vi "FdxCmdBoardControlCvi.vi"(8 "error in":errorcluster, 9 "BoardControlIn (read)":T4 {"Expert4Mode" items=["FDX_EXPERT_MODE", "FDX_DISA_GHOST"]; "Expert3Mode" items=["FDX_EXPERT_MODE", "FDX_DISA_GHOST"]; "Expert2Mode" items=["FDX_EXPERT_MODE", "FDX_DISA_GHOST"]; "Expert1Mode" items=["FDX_EXPERT_MODE", "FDX_DISA_GHOST"]; "Port4SpeedIn" items=["FDX_100MBIT", "FDX_10MBIT", "FDX_AUTO_100MBIT", "FDX_AUTO_10MBIT"]; "Port3SpeedIn" items=["FDX_100MBIT", "FDX_10MBIT", "FDX_AUTO_100MBIT", "FDX_AUTO_10MBIT"]; "Port2SpeedIn" items=["FDX_100MBIT", "FDX_10MBIT", "FDX_AUTO_100MBIT", "FDX_AUTO_10MBIT"]; "Port1SpeedIn" items=["FDX_100MBIT", "FDX_10MBIT", "FDX_AUTO_100MBIT", "FDX_AUTO_10MBIT"]; "Port4ConfigIn" items=["FDX_SINGLE", "FDX_REDUNDANT"]; "Port3ConfigIn" items=["FDX_SINGLE", "FDX_REDUNDANT"]; "Port2ConfigIn" items=["FDX_SINGLE", "FDX_REDUNDANT"]; "Port1ConfigIn" items=["FDX_SINGLE", "FDX_REDUNDANT"]; "Control" items=["FDX_READ", "FDX_WRITE"]}, 11 "InstrumentHandle_board in":u32) -> (0 "error out":errorcluster, 1 "Board Control Out":T6 {"SharedMemFree" format="%x"; "GlobalMemFree" format="%x"; "ExpertMode" items=["FDX_EXPERT_MODE", "FDX_DISA_GHOST"]; "PortGoodLink" items=["FDX_NO_LINK", "FDX_GOOD_LINK"]; "PortSpeed" items=["FDX_100MBIT", "FDX_10MBIT", "FDX_AUTO_100MBIT", "FDX_AUTO_10MBIT"]; "PortConfig" items=["FDX_SINGLE", "FDX_REDUNDANT"]}, 3 "InstrumentHandle_board out":u32)   [LabVIEW 2020, in "AIM664LV.lvlib"]
doc: "This function is used to control the global settings of the board. For the AIM-FDX board this means the organization of the physical ports to logical single or redundant ports."
uses:
  AIM664LV.lvlib
  _controls/port_configuration.ctl
  _controls/port_speed.ctl
  _controls/port_condition.ctl
  _controls/expert_mode.ctl
  AFDX_LibraryAdmin/FdxGlobalDllPath.vi
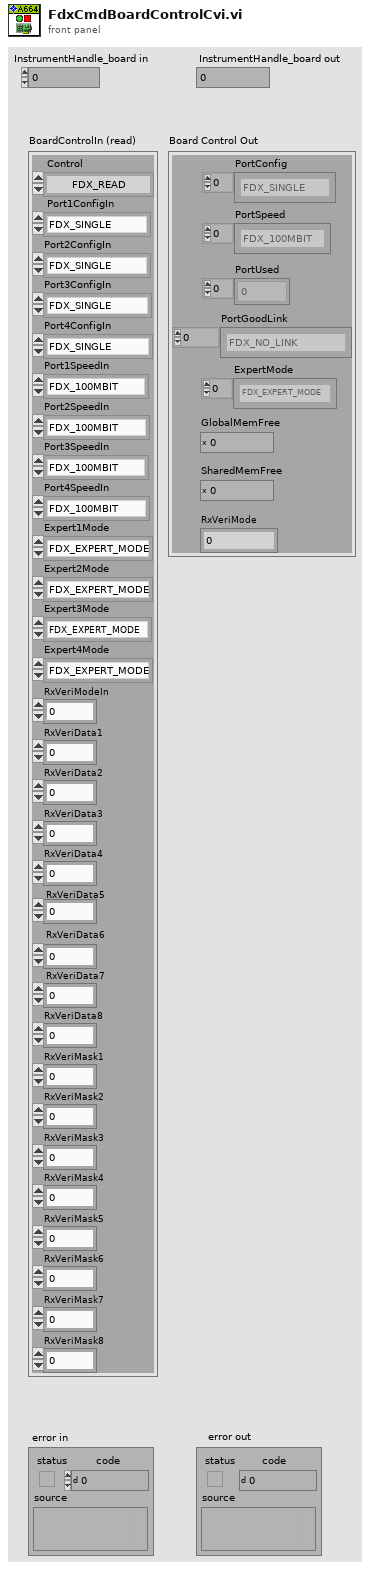
[diagram p1: front panel]
types:
  T1 = typedef "AIM664LV.lvlib/port_configuration.ctl" = u32
  T2 = typedef "AIM664LV.lvlib/port_speed.ctl" = u32
  T3 = typedef "AIM664LV.lvlib/expert_mode.ctl" = u32
  T4 = cluster{"Control":u32, "Port1ConfigIn":T1, "Port2ConfigIn":T1, "Port3ConfigIn":T1, "Port4ConfigIn":T1, "Port1SpeedIn":T2, "Port2SpeedIn":T2, "Port3SpeedIn":T2, "Port4SpeedIn":T2, "Expert1Mode":T3, "Expert2Mode":T3, "Expert3Mode":T3, "Expert4Mode":T3, "RxVeriModeIn":u32, "RxVeriData1":u32, "RxVeriData2":u32, "RxVeriData3":u32, "RxVeriData4":u32, "RxVeriData5":u32, "RxVeriData6":u32, "RxVeriData7":u32, "RxVeriData8":u32, "RxVeriMask1":u32, "RxVeriMask2":u32, "RxVeriMask3":u32, "RxVeriMask4":u32, "RxVeriMask5":u32, "RxVeriMask6":u32, "RxVeriMask7":u32, "RxVeriMask8":u32}
  T5 = typedef "AIM664LV.lvlib/port_condition.ctl" = u32
  T6 = cluster{"PortConfig":T1[], "PortSpeed":T2[], "PortUsed":u32[], "PortGoodLink":T5[], "ExpertMode":T3[], "GlobalMemFree":u32, "SharedMemFree":u32, "RxVeriMode":u32}
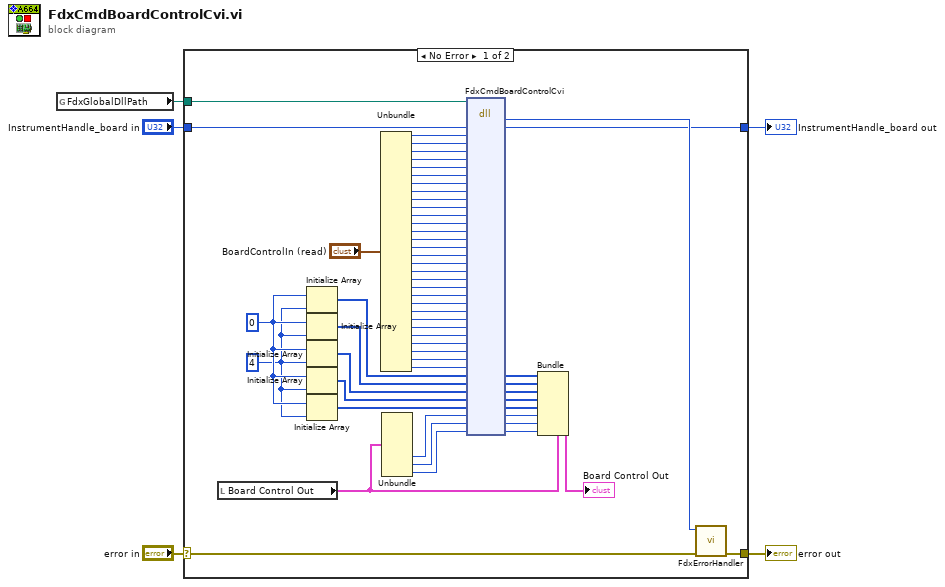
[diagram p0: block diagram]
diagram:
  n1 = global read "FdxGlobalDllPath.vi" "FdxGlobalDllPath"() -> (w3:path)
  n2 = case shown="No Error" "error in" {
    selector: "error in" -> [w62 w64]
    tunnel: [w61 w64] -> w5
    tunnel: w3 -> [w8 _]
    tunnel: "InstrumentHandle_board in" -> [w7 w63]
    tunnel: [w6 w63] -> w1
    frame No Error {
      w49 = 4
      w50 = u32 0
      n3 = local read "Board Control Out"() -> (w9:T6)
      n4 = Initialize Array(w50, w49) -> (w40:u32[])
      n5 = Initialize Array(w50, w49) -> (w39:u32[])
      n6 = Initialize Array(w50, w49) -> (w38:u32[])
      n7 = Initialize Array(w50, w49) -> (w37:u32[])
      n8 = Initialize Array(w50, w49) -> (w36:u32[])
      n9 = Unbundle("BoardControlIn (read)") -> ("Control"=w59:u32, "Port1ConfigIn"=w58:T1, "Port2ConfigIn"=w57:T1, "Port3ConfigIn"=w56:T1, "Port4ConfigIn"=w55:T1, "Port1SpeedIn"=w54:T2, "Port2SpeedIn"=w53:T2, "Port3SpeedIn"=w52:T2, "Port4SpeedIn"=w51:T2, "Expert1Mode"=w48:T3, "Expert2Mode"=w47:T3, "Expert3Mode"=w46:T3, "Expert4Mode"=w41:T3, "RxVeriModeIn"=w44:u32, "RxVeriData1"=w43:u32, "RxVeriData2"=w42:u32, "RxVeriData3"=w29:u32, "RxVeriData4"=w28:u32, "RxVeriData5"=w27:u32, "RxVeriData6"=w26:u32, "RxVeriData7"=w25:u32, "RxVeriData8"=w24:u32, "RxVeriMask1"=w23:u32, "RxVeriMask2"=w22:u32, "RxVeriMask3"=w21:u32, "RxVeriMask4"=w20:u32, "RxVeriMask5"=w19:u32, "RxVeriMask6"=w18:u32, "RxVeriMask7"=w17:u32, "RxVeriMask8"=w16:u32)
      n10 = Unbundle(w9) -> ("GlobalMemFree"=w15:u32, "SharedMemFree"=w14:u32, "RxVeriMode"=w13:u32)  [unwired: 5 out]
      n11 = dll-call lib="aim_fdx.19.dll" fn="FdxCmdBoardControlCvi"(path in=w8, "InstrumentHandle"=w7, "Control"=w59, "Port1ConfigIn"=w58, "Port2ConfigIn"=w57, "Port3ConfigIn"=w56, "Port4ConfigIn"=w55, "Port1SpeedIn"=w54, "Port2SpeedIn"=w53, "Port3SpeedIn"=w52, "Port4SpeedIn"=w51, "Expert1Mode"=w48, "Expert2Mode"=w47, "Expert3Mode"=w46, "Expert4Mode"=w41, "RxVeriModeIn"=w44, "RxVeriData1"=w43, "RxVeriData2"=w42, "RxVeriData3"=w29, "RxVeriData4"=w28, "RxVeriData5"=w27, "RxVeriData6"=w26, "RxVeriData7"=w25, "RxVeriData8"=w24, "RxVeriMask1"=w23, "RxVeriMask2"=w22, "RxVeriMask3"=w21, "RxVeriMask4"=w20, "RxVeriMask5"=w19, "RxVeriMask6"=w18, "RxVeriMask7"=w17, "RxVeriMask8"=w16, "PortConfig"=w40, "PortSpeed"=w39, "PortUsed"=w38, "PortGoodLink"=w37, "ExpertMode"=w36, "GlobalMemFree"=w15, "SharedMemFree"=w14, "RxVeriMode"=w13) -> ("status"=w30:i32, "InstrumentHandle"=w6:u32, "PortConfig"=w32:u32[], "PortSpeed"=w33:u32[], "PortUsed"=w34:u32[], "PortGoodLink"=w31:u32[], "ExpertMode"=w35:u32[], "GlobalMemFree"=w12:u32, "SharedMemFree"=w11:u32, "RxVeriMode"=w10:u32)  [unwired: 32 in, 2 out]
      n12 = Bundle(cluster=w9, "PortConfig"=w32, "PortSpeed"=w33, "PortUsed"=w34, "PortGoodLink"=w31, "ExpertMode"=w35, "GlobalMemFree"=w12, "SharedMemFree"=w11, "RxVeriMode"=w10) -> (→"Board Control Out":T6)
      n13 = call "FdxErrorHandler.vi"("error in"=w62, "AIM Error"=w30) -> ("error out"=w61:errorcluster)  [unwired: 9 in]
    }
    frame Error {
    }
  }
  "error out" <- w5
  "InstrumentHandle_board out" <- w1
